vi "Configure.vi"(8 "error in (no error)":errorcluster) -> (0 "error out":errorcluster, 2 "valid configuration":bool, 3 "config out":T1)   [LabVIEW 2017, in "EmsaDataEventCreator.lvlib"]
uses:
  <vilib>/addons/InsightCM/Devices/Shared/Emsa/EmsaDataEventCreator/EmsaDataEventCreator.lvlib
  <vilib>/addons/InsightCM/Devices/Shared/Emsa/EmsaDataEventCreator/controls/config.ctl
  <vilib>/addons/InsightCM/Devices/Shared/Emsa/EmsaDataEventCreator/controls/DataEventConfig.ctl
  <vilib>/addons/PointValueMap/controls/PointMap.ctl
  <vilib>/addons/InsightCM/Devices/Shared/Emsa/EmsaDataEventCreator/controls/SweepParams.ctl
  <vilib>/addons/InsightCM/Devices/Shared/Emsa/EmsaDataEventCreator/controls/Registry.ctl
  <vilib>/addons/InsightCM/Devices/Shared/Emsa/EmsaDataEventCreator/controls/Registry_Sweep.ctl
  <vilib>/addons/InsightCM/Devices/Shared/Common/DataEvent/controls/DataSetType.ctl
  <vilib>/addons/InsightCM/MessageBus/Base/controls/KeyValuePair.ctl
  <vilib>/addons/InsightCM/Devices/Shared/Common/DataEventCreator/controls/Registry_Trend.ctl
  <vilib>/addons/InsightCM/Utilities/GlobalConfiguration/GlobalConfiguration.lvlib
  <vilib>/addons/PointValueMap/PointValueMap.lvlib
  <vilib>/addons/InsightCM/Devices/Shared/Common/DataEventCreator/DataEventCreator.lvlib
  <vilib>/addons/InsightCM/Devices/Shared/Common/DataEvent/DataEvent.lvlib
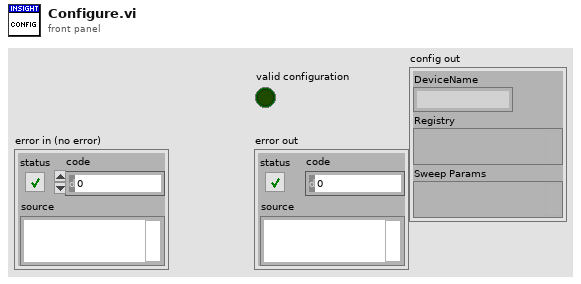
[diagram p1: front panel]
types:
  T1 = typedef "EmsaDataEventCreator.lvlib/config.ctl" = cluster{"DeviceName":string, "Registry":variant, "Sweep Params":variant}
  T2 = typedef "R2_Channel.ctl" = cluster{"Id":string, "DeviceId":string, "Name":string, "ChannelType":string, "HardwareKey":string, "HardwareChannel":string, "DataGroup":string, "Keywords":string[], "EquipmentIds":string[], "Properties":T3[], "Metrics":T4[], "AssetNodeId":string, "MeasType":string, "AssetName":string}
  T3 = typedef "KeyValuePair.ctl" = cluster{"Key":string, "Value":string}
  T4 = typedef "Metric.ctl" = cluster{"Id":string, "Name":string, "Unit":string, "Properties":T3[], "MetricDefinitionInstanceId":string}
  T5 = typedef "R2_Device.ctl" = cluster{"Id":string, "Name":string, "DeviceType":string, "HardwareName":string, "IpAddress":string, "HardwareInfo":T3[], "ApplicationType":string, "ApplicationVersion":string, "EquipmentIds":string[], "ConfigurationVersion":string, "State":T6, "Properties":T3[], "DataGroups":T7[], "BurstModeTrigger":T11}
  T6 = typedef "DeviceState.ctl" = cluster{"Disabled":bool}
  T7 = typedef "R2_DataGroup.ctl" = cluster{"Name":string, "OperatingStates":T8[], "Properties":T3[], "EquipmentIds":string[], "AssetNodeId":string}
  T8 = typedef "OperatingState.ctl" = cluster{"Name":string, "Properties":T3[], "Triggers":T9[]}
  T9 = typedef "Trigger.ctl" = cluster{"Type":string, "Expression":string, "Conditions":T10[]}
  T10 = typedef "Condition.ctl" = cluster{"Source":string, "Type":string, "Operator":string, "CompareTo":string, "DwellSeconds":dbl}
  T11 = typedef "BurstModeTrigger.ctl" = cluster{"Trigger":T9, "SampleRate":string, "AcquisitionLength":string}
  T12 = typedef "EmsaDataEventCreator.lvlib/Registry.ctl" = cluster{"Sweep Registry":T13[], "Trend Points":T15[], "AssetNodeMap":variant}
  T13 = typedef "EmsaDataEventCreator.lvlib/Registry_Sweep.ctl" = cluster{"Name":string, "DataSetType":T14, "Properties":T3[]}
  T14 = typedef "DataEvent.lvlib/DataSetType.ctl" = enum16{"Waveform", "SpeedProfile", "ThermalImage", "EmsaSweep"}
  T15 = typedef "DataEventCreator.lvlib/Registry_Trend.ctl" = cluster{"TrendPointId":string, "DataSetName":string, "HighRate":bool, "Always Send":bool}
  T16 = typedef "EmsaDataEventCreator.lvlib/DataEventConfig.ctl" = cluster{"OpState":string, "ExitOpState":bool, "Reason":string, "StreamId":string, "Map":T17, "DataSetIds":variant, "IncludeWaveforms":bool, "TrendPointsOnly":bool, "Sweep Params":T18}
  T17 = typedef "PointValueMap.lvlib/PointMap.ctl" = refnum<data-value>
  T18 = typedef "EmsaDataEventCreator.lvlib/SweepParams.ctl" = cluster{"CollectOnEnter":bool, "CollectOnExit":bool}
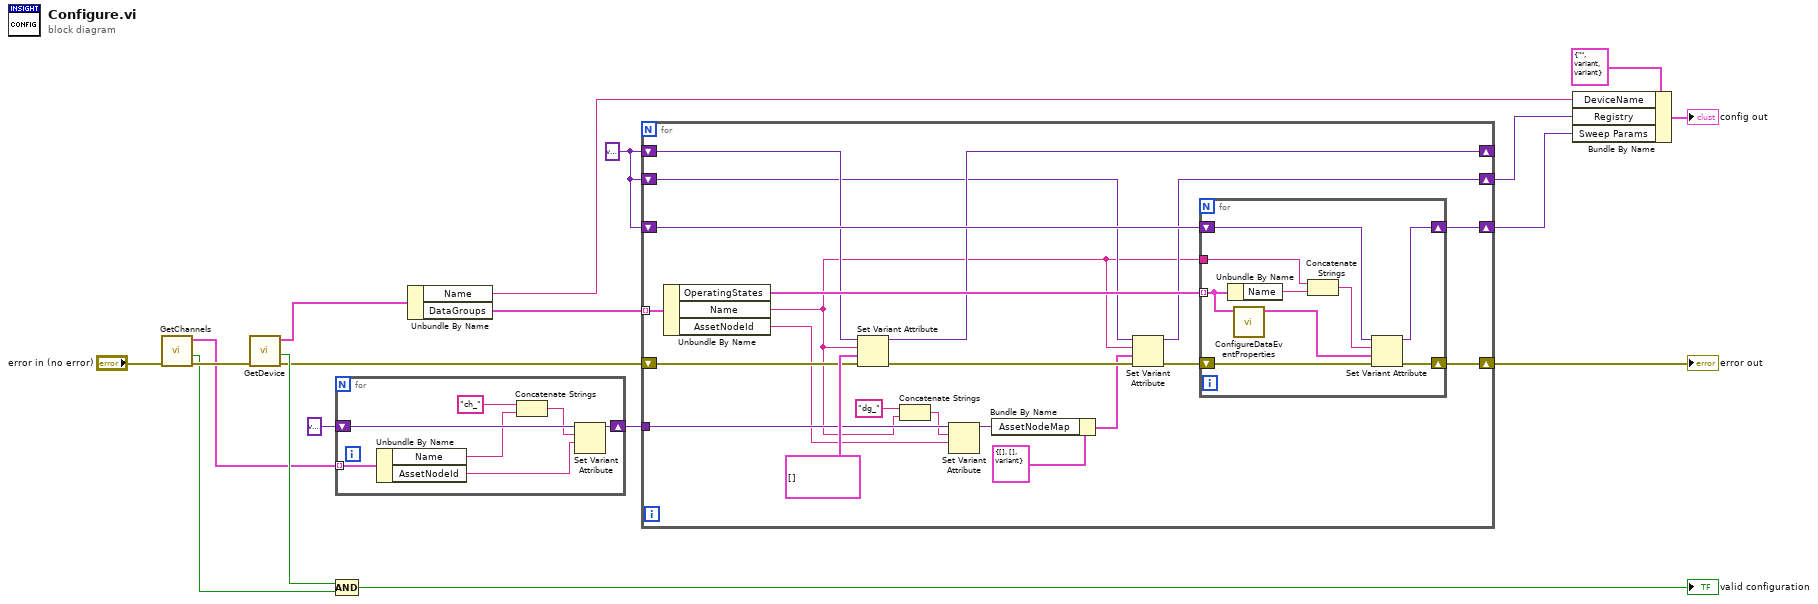
[diagram p0: block diagram]
diagram:
  w9 = variant
  n1 = call <vilib>:"GetChannels.vi"("error in (no error)"="error in (no error)") -> ("error out"=w12:errorcluster, "found"=w11:bool, "channels"=w6:T2[])  [unwired: 8 in]
  n2 = call <vilib>:"GetDevice.vi"("error in (no error)"=w12) -> ("error out"=w10:errorcluster, "found"=w15:bool, "device configuration"=w17:T5)  [unwired: 8 in]
  n3 = for {
    shift-right: [w23] -> w5
    shift-left: variant -> [w24]
    tunnel: w6 -> [w25] mode=indexing
    n4 = Unbundle By Name(w25) -> ("Name"=w20:string, "AssetNodeId"=w22:string)
    n5 = Concatenate Strings("ch_" ("string"), w20) -> (w19:string)
    n6 = Set Variant Attribute(Variant=w24, name=w19, value=w22) -> (Variant out=w23:variant)  [unwired: 1 in, 2 out]
  }
  n7 = Compound Arithmetic op=AND(w15, w11) -> (→"valid configuration":bool)
  n8 = Unbundle By Name(w17) -> ("Name"=w13:string, "DataGroups"=w18:T7[])
  n9 = for {
    shift-right: [w36] -> w16
    shift-left: w10 -> [w38]
    tunnel: w18 -> [w45] mode=indexing
    shift-right: [w42] -> w2
    shift-left: w9 -> [w44]
    shift-right: [w40] -> _
    shift-left: w9 -> [w41]
    shift-right: [w34] -> w8
    shift-left: w9 -> [w35]
    tunnel: w5 -> [w31]
    n10 = Unbundle By Name(w45) -> ("OperatingStates"=w43:T8[], "Name"=w27:string, "AssetNodeId"=w30:string)
    n11 = Set Variant Attribute(Variant=w41, name=w27, value=T16[] [], error in=w38) -> (Variant out=w40:variant, error out=w37:errorcluster)  [unwired: 1 out]
    n12 = Concatenate Strings("dg_" ("string"), w27) -> (w26:string)
    n13 = Set Variant Attribute(Variant=w31, name=w26, value=w30) -> (Variant out=w32:variant)  [unwired: 1 in, 2 out]
    n14 = Bundle By Name(cluster=T12 {"Sweep Registry"=[], "Trend Points"=[], "AssetNodeMap"=variant} ("Registry"), "AssetNodeMap"=w32) -> (w33:T12)
    n15 = Set Variant Attribute(Variant=w35, name=w27, value=w33, error in=w37) -> (Variant out=w34:variant, error out=w36:errorcluster)  [unwired: 1 out]
    n16 = for {
      shift-right: [w47] -> _
      shift-left: w36 -> [w54]
      shift-right: [w52] -> w42
      shift-left: w44 -> [w53]
      tunnel: w27 -> [w50]
      tunnel: w43 -> [w48] mode=indexing
      n17 = Unbundle By Name(w48) -> ("Name"=w51:string)
      n18 = call <vilib>:"ConfigureDataEventProperties.vi"("operating state"=w48) -> ("Sweep Param"=w46:T18)  [unwired: 10 in]
      n19 = Concatenate Strings(w50, w51) -> (w49:string)
      n20 = Set Variant Attribute(Variant=w53, name=w49, value=w46, error in=w54) -> (Variant out=w52:variant, error out=w47:errorcluster)  [unwired: 1 out]
    }
  }
  "error out" <- w16
  n21 = Bundle By Name(cluster=T1 {"DeviceName"="", "Registry"=variant, "Sweep Params"=variant} ("config"), "DeviceName"=w13, "Registry"=w8, "Sweep Params"=w2) -> (→"config out":T1)
